vi "DSF.Shared.Timing.Get Offset.vi"(11 "Timing in":refnum<class "DSF.Shared.Timing.lvclass">) -> (2 "Offset":T1, 3 "Timing out":refnum<class "DSF.Shared.Timing.lvclass">)   [LabVIEW 2016, in "DSF.Shared.lvlib" / "DSF.Shared.Timing.lvclass"]
uses:
  DSF.Shared.Timing.lvclass
  Typedefs/DSF.Shared.Typedefs.Scalars.Offset.ctl
  DSF.Shared.Timing.lvclass/DSF.Shared.Timing.ctl
  DSF.Shared.lvlib
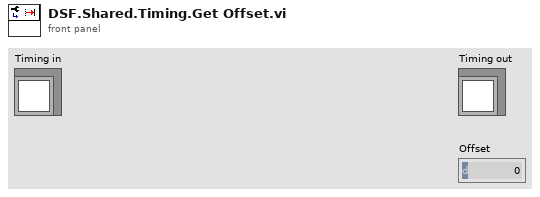
[diagram p1: front panel]
types:
  T1 = typedef "DSF.Shared.lvlib/DSF.Shared.Typedefs.Scalars.Offset.ctl" = u64
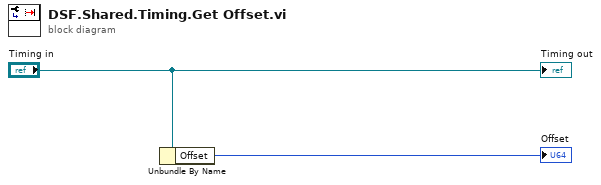
[diagram p0: block diagram]
diagram:
  n1 = Unbundle By Name("Timing in") -> ("Offset"=→"Offset":T1)
  "Timing out" <- "Timing in"
